vi "Game_guessLetter.vi"(8 "error in (no error)":errorcluster, 9 "guess":string, 10 "Solution":string, 11 "Puzzle":string) -> (0 "error out":errorcluster, 1 "Letters Found":i32, 2 "Solution OUT":string, 3 "Puzzle OUT":string)   [LabVIEW 2020]
uses:
  <userlib>/_OpenG.lib/array/array.llb/Filter 1D Array with Scalar (U8)__ogtk.vi
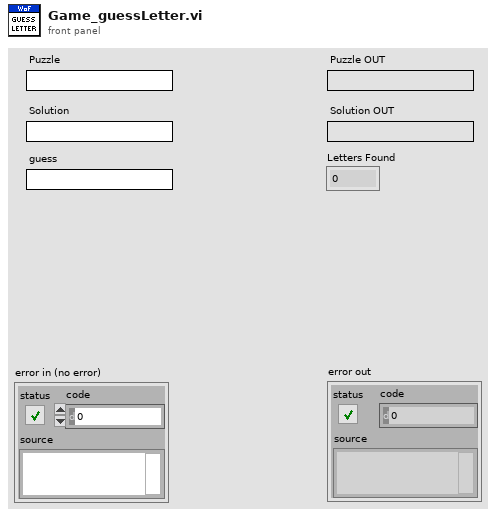
[diagram p1: front panel]
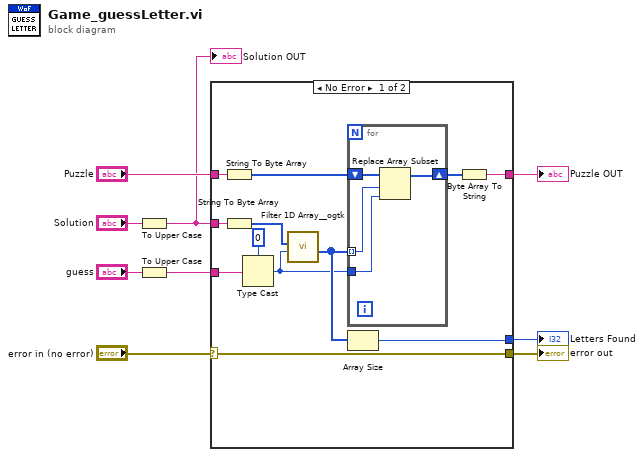
[diagram p0: block diagram]
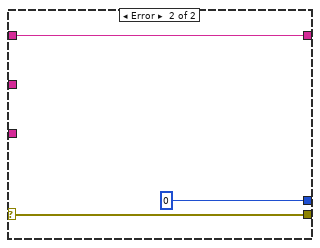
[diagram p2: hidden frame]
diagram:
  n1 = To Upper Case(1:"Solution") -> (0:w3:string)
  "Solution OUT" <- w3
  n2 = To Upper Case(1:"guess") -> (0:w2:string)
  n3 = case shown="No Error" "error in (no error)" {
    selector: "error in (no error)" -> [w17 w27]
    tunnel: w2 -> [w18 _]
    tunnel: w3 -> [w21 _]
    tunnel: "Puzzle" -> [w13 w28]
    tunnel: [w10 w28] -> w5
    tunnel: [w17 w27] -> w4
    tunnel: [w15 0] -> w1
    frame No Error {
      n4 = String To Byte Array(string=w13) -> (unsigned byte array=w12:u8[])
      n5 = String To Byte Array(string=w21) -> (unsigned byte array=w19:u8[])
      n6 = Type Cast(type=u8 0, x=w18) -> (*(type *) &x=w14:u8)
      n7 = call-poly <userlib>:"Filter 1D Array__ogtk.vi"("items to filter"=w14, "array"=w19) -> ("filtered item indices"=w16:i32[])  [unwired: 4 in, 1 out]
      n8 = for {
        tunnel: w16 -> [w23] mode=indexing
        tunnel: w14 -> [w22]
        shift-right: [w24] -> w11
        shift-left: w12 -> [w25]
        n9 = Replace Array Subset(array=w25, new element=w22, index=w23) -> (w24:u8[])
      }
      n10 = Array Size(array=w16) -> (size(s)=w15:i32)
      n11 = Byte Array To String(unsigned byte array=w11) -> (string=w10:string)
    }
    frame Error {
    }
  }
  "error out" <- w4
  "Puzzle OUT" <- w5
  "Letters Found" <- w1
